vi "Example - Simple.vi"() -> ()   [LabVIEW 2017]
uses:
  Timer_class/Timer.lvclass
panel:
  out "Timer Time (min)":dbl
  out "Timer Time (s)":dbl
  out "Timer Time (ms)":u32
  out "Timer is Timing":bool
  in  "Quit Program":bool
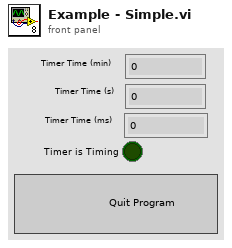
[diagram p1: front panel]
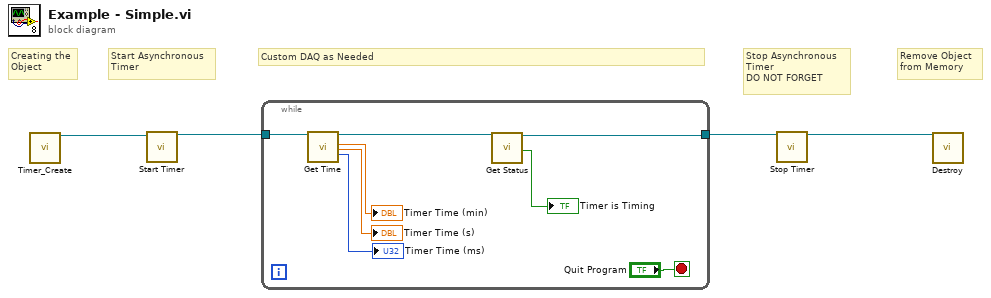
[diagram p0: block diagram]
diagram:
  # "Creating the\nObject"
  # "Start Asynchronous\nTimer"
  # "Custom DAQ as Needed"
  # "Remove Object\nfrom Memory"
  # "Stop Asynchronous\nTimer\nDO NOT FORGET"
  n1 = call "Timer_Create.vi"() -> ("reference out"=w4:refnum<class "Timer.lvclass">)  [unwired: 18 in, 1 out]
  n2 = call-dynamic "Start Timer.vi"("reference in"=w4) -> ("reference out"=w3:refnum<class "Timer.lvclass">)  [unwired: 17 in, 1 out]
  n3 = while {
    tunnel: w3 -> [w10]
    tunnel: [w8] -> w2
    stop <- "Quit Program" stop-if-true
    n4 = call-dynamic "Get Time.vi"("reference in"=w10) -> ("reference out"=w9:refnum<class "Timer.lvclass">, "Timer Time (min)"=→"Timer Time (min)":dbl, "Timer Time (s)"=→"Timer Time (s)":dbl, "Timer Time (ms)"=→"Timer Time (ms)":u32)  [unwired: 14 in, 1 out]
    n5 = call-dynamic "Get Status.vi"("reference in"=w9) -> ("reference out"=w8:refnum<class "Timer.lvclass">, "Timer is Timing"=→"Timer is Timing":bool)  [unwired: 16 in, 1 out]
  }
  n6 = call-dynamic "Stop Timer.vi"("reference in"=w2) -> ("reference out"=w1:refnum<class "Timer.lvclass">)  [unwired: 14 in, 4 out]
  n7 = call-dynamic "Destroy.vi"("reference in"=w1) -> ()  [unwired: 17 in, 2 out]
